vi "smsEnviado.vi"   [LabVIEW 2012]
panel:
  # "SMS enviado"
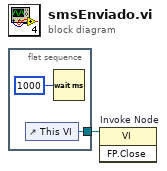
[diagram p0: block diagram]
diagram:
  n1 = flat-sequence {
    tunnel: [w2] -> w1
    frame #0 {
      n2 = control-ref of="This VI"() -> (w2:refnum<vi>)
      n3 = Wait (ms)(milliseconds to wait=u32 1000) -> ()  [unwired: 1 out]
    }
  }
  n4 = invoke on="Invoke Node" class="VI" method="FP.Close"(reference=w1) -> ()  [unwired: 2 in, 3 out]
